vi "Auto 2.vi"   [LabVIEW 2014]
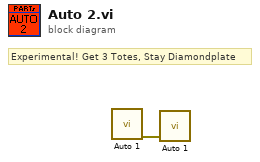
[diagram p0: block diagram]
diagram:
  # "Experimental! Get 3 Totes, Stay Diamondplate"
  n1 = call "Auto 1.vi"() -> ("Error Out"=w1:errorcluster)  [unwired: 11 in]
  n2 = call "Auto 1.vi"("Error In"=w1) -> ()  [unwired: 10 in, 1 out]
